vi "PCO_SetImageTransferMode.vi"(8 "error in (no error)":errorcluster {"code" format="%x"}, 10 "param":T1 {"wMode" items=["IMAGE_TRANSFER_MODE_STANDARD"=0, "IMAGE_TRANSFER_MODE_SCALED_XY_8BIT"=1, "IMAGE_TRANSFER_MODE_CUTOUT_XY_8BIT"=2, "IMAGE_TRANSFER_MODE_FULL_RGB_24BIT"=3, "IMAGE_TRANSFER_MODE_BIN_SCALED_8BIT_BW"=4, "IMAGE_TRANSFER_MODE_BIN_SCALED_8BIT_COLOR"=5, "IMAGE_TRANSFER_MODE_TEST_ONLY"=32768]}, 11 "ph":u64) -> (0 "error out":errorcluster {"code" format="%x"}, 2 "ErrorMessage":i32 format="%x", 3 "ph out":u64)   [LabVIEW 2019, in "SDK.lvlib" / "SpecialCommandsDimax.lvlib"]
doc: "<b>Description:</b>\nThis function does set the scaled image transfer mode of the camera. The image transfer mode can be used to transfer scaled images from the internal memory of the camera. With scaled image transfer the amount of data, which must be transferred for one image, is reduced and therefore the image display frequency can be enhanced. An application can use this mode for display of thumbnails or faster image preview, when camera setup is performed e.g. adjust and focus the camera lens.\nThe IMAGE_TRANSFER_MODE_PARAM structure must be filled with appropriate values.\nBecause scaled image transfer mode is a special mode inside the camera the size parameters must be set to the original camera recording size for the image allocation and acquisition functions like PCO_AllocateBuffer, PCO_GetImageEx or PCO_AddBufferEx.\nWhen any size related camera settings are changed the PCO_SetImageTransferMode has to be called again in order to correctly calculate the transferred amount of data. Also when reading images from different Camera RAM segments, which have different image sizes, the PCO_SetImageTransferMode has to be called after selecting another segment and before reading the images.\nBefore an application is closed the scaled image transfer mode must be reset to standard mode.\n\n<b>Supported camera type:</b>\npco.dimax with GigE or USB interface\n\n<b>Descriptor dependency:</b>\nNone"
uses:
  SpecialCommandsDimax.lvlib
  Structures/Structures.lvlib
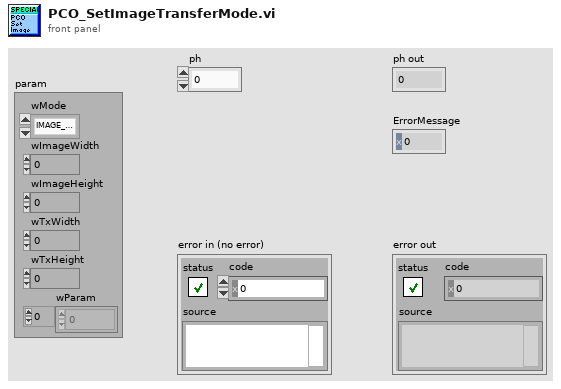
[diagram p1: front panel]
types:
  T1 = cluster{"wMode":u16, "wImageWidth":u16, "wImageHeight":u16, "wTxWidth":u16, "wTxHeight":u16, "wParam":u16[]}
  T2 = cluster{"wSize":u16, "wMode":u16, "wImageWidth":u16, "wImageHeight":u16, "wTxWidth":u16, "wTxHeight":u16, "wParam":cluster{u16, u16, u16, u16, u16, u16, u16, u16}, "ZZwDummy":cluster{u16, u16, u16, u16, u16, u16, u16, u16, u16, u16}}
  T3 = cluster{u16, u16, u16, u16, u16, u16, u16, u16, u16, u16}
  T4 = cluster{"wParam[0]":u16, "wParam[1]":u16, "wParam[2]":u16, "wParam[3]":u16, "wParam[4]":u16, "wParam[5]":u16, "wParam[6]":u16, "wParam[7]":u16}
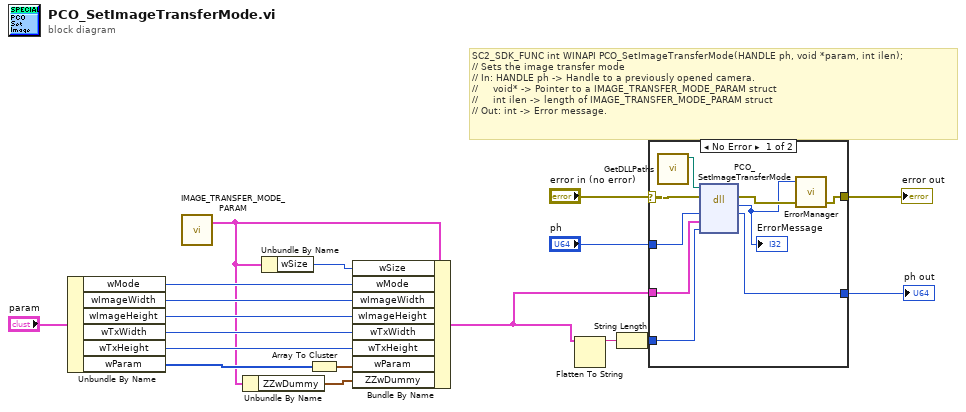
[diagram p0: block diagram]
diagram:
  # "SC2_SDK_FUNC int WINAPI PCO_SetImageTransferMode(HANDLE ph, void *param, int ilen);\n// Sets the image transfer mode\n// In: HANDLE ph -> Handle to a previously opened camera.\n//     void* -> Pointer to a IMAGE_TRANSFER_MODE_PARAM struct\n//     int ilen -> length of IMAGE_TRANSFER_MODE_PARAM struct\n// Out: int -> Error message."
  n1 = Unbundle By Name("param") -> ("wMode"=w13:u16, "wImageWidth"=w12:u16, "wImageHeight"=w11:u16, "wTxWidth"=w10:u16, "wTxHeight"=w9:u16, "wParam"=w8:u16[])
  n2 = call "IMAGE_TRANSFER_MODE_PARAM.vi"() -> ("IMAGE_TRANSFER_MODE_PARAM_RAW"=w5:T2)  [unwired: 4 in, 3 out]
  n3 = Unbundle By Name(w5) -> ("ZZwDummy"=w6:T3)
  n4 = Unbundle By Name(w5) -> ("wSize"=w4:u16)
  n5 = Array To Cluster(array=w8) -> (cluster=w7:T4)
  n6 = Bundle By Name(cluster=w5, "wSize"=w4, "wMode"=w13, "wImageWidth"=w12, "wImageHeight"=w11, "wTxWidth"=w10, "wTxHeight"=w9, "wParam"=w7, "ZZwDummy"=w6) -> (w2:T2)
  n7 = Flatten To String(anything=w2) -> (data string=w3:string)  [unwired: 3 in, 2 out]
  n8 = String Length(string=w3) -> (length=w1:i32)
  n9 = case shown="No Error" "error in (no error)" {
    selector: "error in (no error)" -> [w23 w29]
    tunnel: "ph" -> [w27 w28]
    tunnel: [w26 w28] -> w17
    tunnel: w2 -> [w25 _]
    tunnel: w1 -> [w24 _]
    tunnel: [w21 w29] -> w16
    frame No Error {
      n10 = call "GetDLLPaths.vi"() -> ("SC2_Cam_Path"=w19:path)  [unwired: 8 in, 3 out]
      n11 = dll-call lib="?" fn="PCO_SetImageTransferMode"(path in=w19, error in=w23, "ph"=w27, "param"=w25, "ilen"=w24) -> (error out=w22:errorcluster, "return type"=w20:i32, "ph"=w26:u64)  [unwired: 3 in, 1 out]
      "ErrorMessage" <- w20
      n12 = call "ErrorManager.vi"("error in (no error)"=w22, "error code"=w20) -> ("error out"=w21:errorcluster)  [unwired: 2 in, 1 out]
    }
    frame Error {
    }
  }
  "ph out" <- w17
  "error out" <- w16
